vi "Get Variable From Devices.vi"() -> ()   [LabVIEW 2020]
panel:
  in  "Tab Control":enum32{"MAIN", "DEVICE TYPE LIST"}(tab)
  out "Device name":string
  out "error out":errorcluster
  out "timed \nout":bool
  out "variable value":string
  in  "Variable Name":string
  out "Results":string[][](table)
  in  "Search Element":string
  in  "Search":bool
  in  "exit":bool
  in  "GO":bool
  out "Search Result":string[](array[string])
  out "Progress Bar":u8(slide) max=141 scale=0.0..141.0
  in  "Device Types":string[](array[string])=["Point Grey Camera", "", " ", " ", "", "", "", "", "", ""]
  in  "Use All":bool caption="Use Premade List of All Camera Device Types"
  # "VARIABLE  SEARCH"
  # "OR"
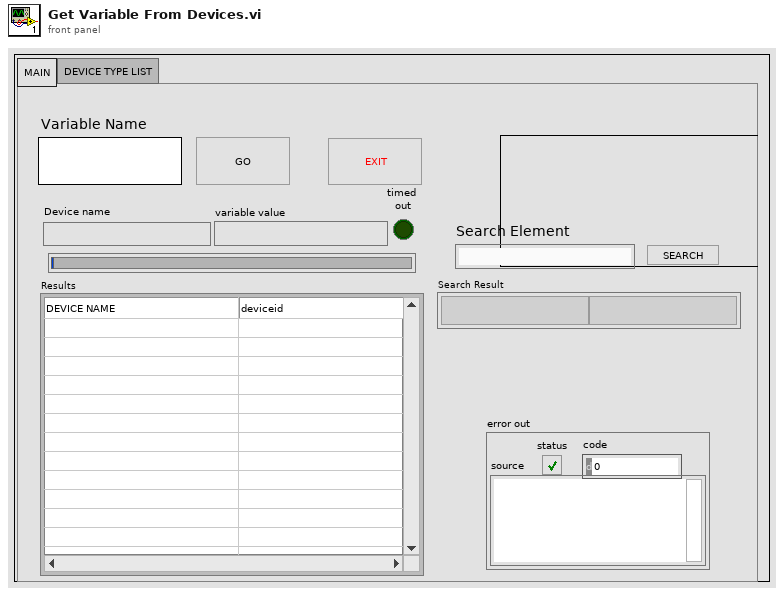
[diagram p1: front panel]
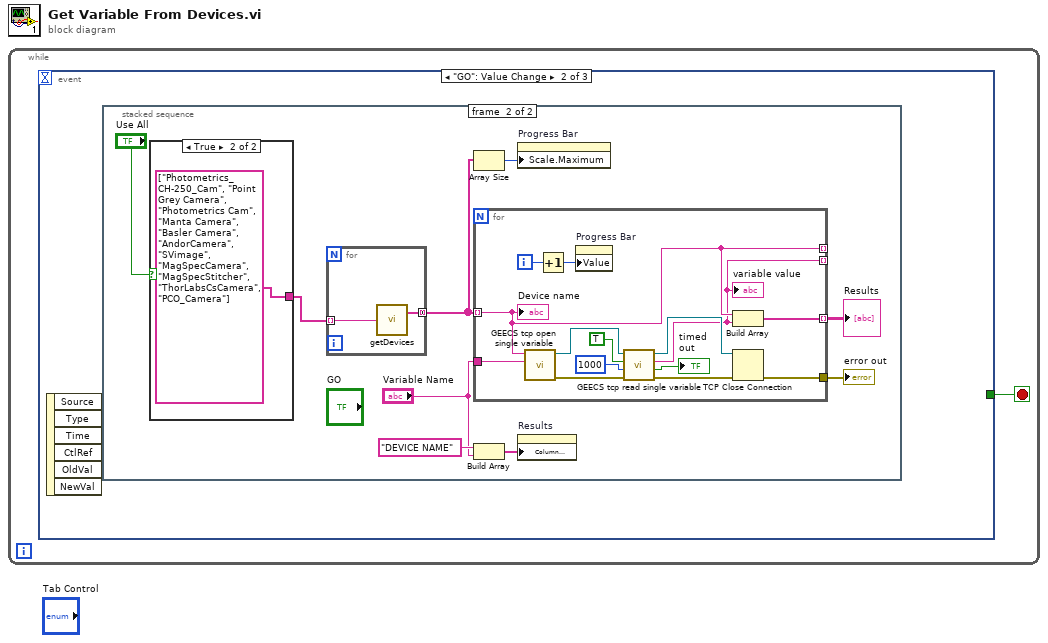
[diagram p0: block diagram]
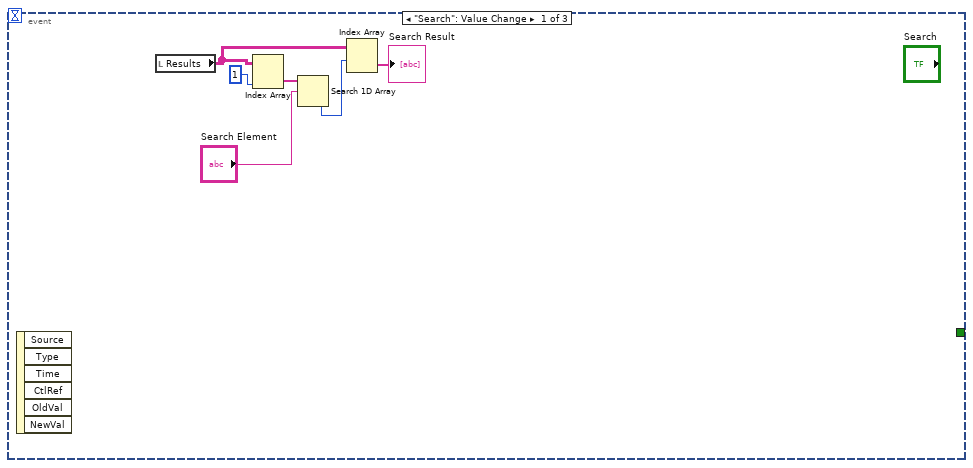
[diagram p2: hidden frame]
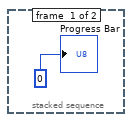
[diagram p3: hidden frame]
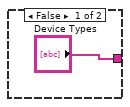
[diagram p4: hidden frame]
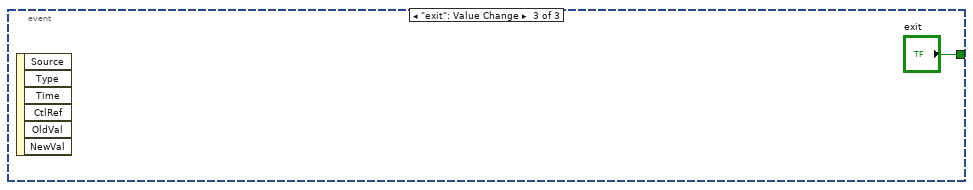
[diagram p5: hidden frame]
diagram:
  n1 = while {
    stop <- w1 stop-if-true
    n2 = event shown="[1] \"GO\": Value Change" {
      selector: _ -> [_ _ _]
      dyn-events: _ -> [_ _ _]
      timeout: _ -> [_ _ _]
      tunnel: [_ _ "exit"] -> w1
      event "Search": Value Change {
        n3 = event-data() -> ()  [unwired: 1 in, 6 out]
        n4 = local read "Results"() -> (w2:string[][])
        n5 = Index Array(array=w2, index (col)=1 ("disabled index (col)")) -> (element=w6:string[])  [unwired: 1 in]
        n6 = Search 1D Array(1D array=w6, element="Search Element") -> (index of element=w4:i32)  [unwired: 1 in]
        n7 = Index Array(array=w2, index (row)=w4) -> (element=→"Search Result":string[])  [unwired: 1 in]
      }
      event "GO": Value Change {
        n8 = event-data() -> ()  [unwired: 1 in, 6 out]
        n9 = stacked-sequence {
          frame #0 {
            "Progress Bar" <- u8 0 ("Progress Bar")
          }
          frame #1 {
            n10 = case shown="True" "Use All" {
              tunnel: ["Device Types" string[] ["Photometrics_CH-250_Cam", "Point Grey Camera", "Photometrics Cam", "Manta Camera", "Basler Camera", "AndorCamera", "SVimage", "MagSpecCamera", "MagSpecStitcher", "ThorLabsCsCamera", "PCO_Camera"] ("DeviceTypeNames")] -> w16
              frame False {
              }
              frame True {
              }
            }
            n11 = for {
              tunnel: [w35] -> w11 mode=concatenating
              tunnel: w16 -> [w34] mode=indexing
              n12 = call "getDevices.vi"("Device Class"=w34) -> ("All Devices"=w35:string[])  [unwired: 1 out]
            }
            n13 = Array Size(array=w11) -> (size(s)=w10:i32)
            n14 = for {
              tunnel: [w33] -> w17
              tunnel: w11 -> [w25] mode=indexing
              tunnel: [w25] -> _ mode=indexing
              tunnel: [w24] -> _ mode=indexing
              tunnel: [w23] -> w15 mode=indexing
              tunnel: "Variable Name" -> [w22]
              i -> [w21]
              n15 = call "GEECS tcp open single variable.vi"("Variable name"=w22, "Device name"=w25) -> ("error out"=w29:errorcluster, "TCP Network Connection out"=w30:refnum<k5>)  [unwired: 7 in, 1 out]
              n16 = Increment(x=w21) -> (x+1=w20:i32)
              n17 = property on="Progress Bar" class="Slide (strict)"("Value"=w20) -> ()  [unwired: 2 in, 2 out]
              n18 = call "GEECS tcp read single variable.vi"("error in (no error)"=w29, "timeout ms (2000)"=1000, "clear buffer after read"=TRUE, "TCP Network Connection in"=w30) -> ("error out"=w27:errorcluster, "timed out"=→"timed \nout":bool, "variable value"=w24:string, "TCP Network Connection out"=w28:refnum<k5>)  [unwired: 4 in]
              "variable value" <- w24
              n19 = Build Array(w25, w24) -> (w23:string[])
              n20 = TCP Close Connection(connection ID=w28, error in (no error)=w27) -> (error out=w33:errorcluster)  [unwired: 1 in, 1 out]
              "Device name" <- w25
            }
            "error out" <- w17
            "Results" <- w15
            n21 = Build Array("DEVICE NAME", "Variable Name") -> (w14:string[])
            n22 = property on="Progress Bar" class="Slide (strict)"("Scale.Maximum"=w10) -> ()  [unwired: 2 in, 2 out]
            n23 = property on="Results" class="Tbl (strict)"("Column Headers[]"=w14) -> ()  [unwired: 2 in, 2 out]
          }
        }
      }
      event "exit": Value Change {
        n24 = event-data() -> ()  [unwired: 1 in, 6 out]
      }
    }
  }
